vi "Check Empty JSON Array.vi"(11 "JSON":string) -> (3 "JSON":string)   [LabVIEW 2020, in "wamplv.lvlib" / "WAMP Client.lvclass"]
uses:
  WAMP Client.lvclass
  WAMP Client.lvclass/WAMP Client.ctl
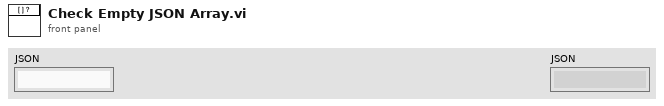
[diagram p1: front panel]
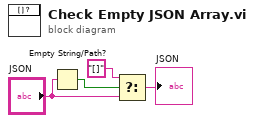
[diagram p0: block diagram]
diagram:
  n1 = Empty String/Path?(string/path="JSON") -> (empty?=w4:bool)
  n2 = Select(t="[]" ("f"), s=w4, f="JSON") -> (s? t:f=→"JSON":string)
